vi "Get control name.vi"(1 "Control ref in":refnum<vi>) -> (0 "Control name out":string)   [LabVIEW 2018]
doc: "By default returns the label text.\n\nThis VI is used internally to determine how controls should be named specifically for the \"Update control(s)\" event in the Model loop.\n\nIf there is ever a case where the label text should not be the name it's known by, add an exception here."
uses:
  <vilib>/Utility/error.llb/Clear Errors.vi
  <userlib>/nLight Error Handling/Log any errors.vi
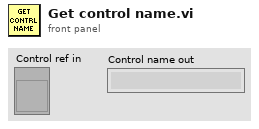
[diagram p1: front panel]
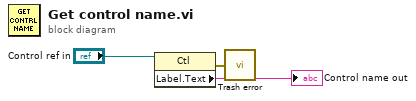
[diagram p0: block diagram]
diagram:
  n1 = property class="Ctl"(reference="Control ref in") -> (error out=w1:errorcluster, "Label.Text"=→"Control name out":string)  [unwired: 1 in, 1 out]
  n2 = call <userlib>:"Trash error.vi"("error in"=w1) -> ()  [unwired: 15 in]
